vi "Kundt's Tube.vi"() -> ()   [LabVIEW 2015]
panel:
  in  "Amplitude":dbl
  in  "stop":bool
  out "RMS":dbl
  out "Waveform Graph":dynamicdata(graph)
  in  "Tab Control":enum32{"Sweep", "Single"}(tab)
  in  "Dwell Time (s)":dbl
  in  "Frequency (Hz)":dbl
  out "Gain vs. Frequency":cluster{"X":dbl, "Y":dbl}[](graph)
  in  "Cluster 3":T1
  in  "Cluster":T2
  # "This will sweep from Min to Max, \nPausing for the dwell time after \neach increment."
  # "Generates a static frequency."
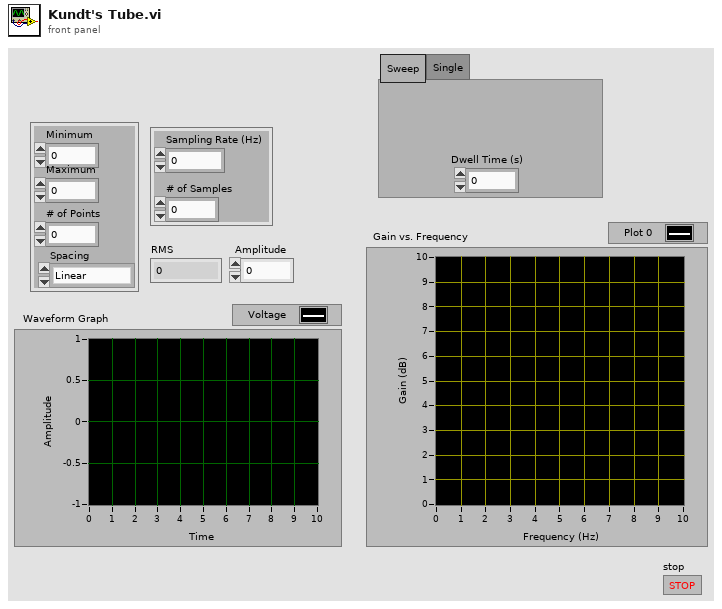
[diagram p1: front panel]
types:
  T1 = cluster{"Sampling Rate (Hz)":dbl, "# of Samples":i32}
  T2 = cluster{"Minimum":dbl, "Maximum":dbl, "# of Points":dbl, "Spacing":enum16{"Linear", "Logarithmic"}}
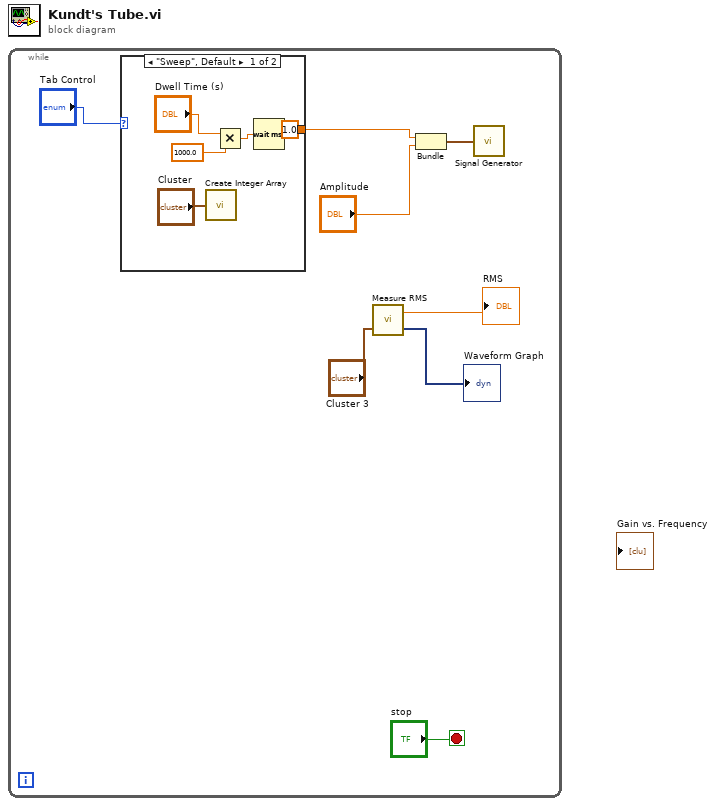
[diagram p0: block diagram]
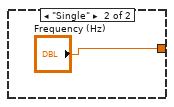
[diagram p2: hidden frame]
diagram:
  n1 = while {
    stop <- "stop" stop-if-true
    n2 = case shown="\"Sweep\", Default" "Tab Control" {
      tunnel: [1.0 ("Frequency (Hz)") "Frequency (Hz)"] -> w3
      frame "Sweep", Default {
        n3 = call "Create Integer Array.vi"("Cluster"="Cluster") -> ()  [unwired: 1 out]
        n4 = Multiply(x="Dwell Time (s)", y=1000.0) -> (x*y=w11:dbl)
        n5 = Wait (ms)(milliseconds to wait=w11) -> ()  [unwired: 1 out]
      }
      frame "Single" {
      }
    }
    n6 = call "Measure RMS.vi"("Cluster"="Cluster 3") -> ("Waveform Graph"=→"Waveform Graph":dynamicdata, "RMS"=→"RMS":dbl)  [unwired: 1 in]
    n7 = Bundle("Frequency (Hz)"=w3, "Amplitude"="Amplitude") -> (w1:cluster{"Frequency (Hz)":dbl, "Amplitude":dbl})  [unwired: 1 in]
    n8 = call "Signal Generator.vi"("Cluster"=w1) -> ()
  }
